vi "simplePID core.vi"(0 "errors":T2 {"error" step=0.125}, 1 "reset? (F)":bool, 7 "manual control":T6, 11 "state in":T3, 12 "gains":T4 {"filter coefficient" min=0 max=1; "proportional gain" step=0.125}, 13 "output range":T5={"output high (Inf)"=inf, "output low (-Inf)"=-inf}) -> (4 "output":sgl, 6 "error":sgl, 8 "actions":T1, 15 "state out":T3)   [LabVIEW 2020]
uses:
  Typedef/niFpgaPID_ManualControl.ctl
  Typedef/niFpgaPID_OutputRange.ctl
  Typedef/niFpgaPID_PIDGains.ctl
  <vilib>/rvi/Analysis/control/PID/Typedef/niFpgaPID_PIDState.ctl
  <vilib>/rvi/Analysis/control/PID/Typedef/niFpgaPID_PIDErrors.ctl
  Typedef/niFpgaPID_PIDActions.ctl
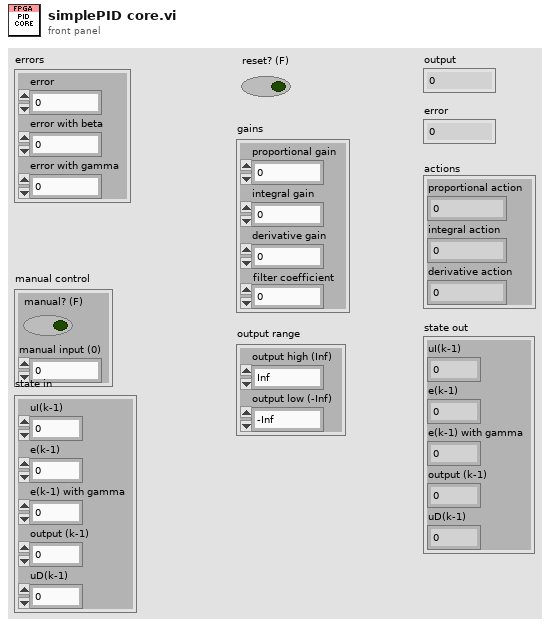
[diagram p1: front panel]
types:
  T1 = typedef "niFpgaPID_PIDActions.ctl" = cluster{"proportional action":sgl, "integral action":sgl, "derivative action":sgl}
  T2 = typedef "niFpgaPID_PIDErrors.ctl" = cluster{"error":sgl, "error with beta":sgl, "error with gamma":sgl}
  T3 = typedef "niFpgaPID_PIDState.ctl" = cluster{"uI(k-1)":sgl, "e(k-1)":sgl, "e(k-1) with gamma":sgl, "output (k-1)":sgl, "uD(k-1)":sgl}
  T4 = typedef "niFpgaPID_PIDGains.ctl" = cluster{"proportional gain":sgl, "integral gain":sgl, "derivative gain":sgl, "filter coefficient":sgl}
  T5 = typedef "niFpgaPID_OutputRange.ctl" = cluster{"output high (Inf)":sgl, "output low (-Inf)":sgl}
  T6 = typedef "niFpgaPID_ManualControl.ctl" = cluster{"manual? (F)":bool, "manual input (0)":sgl}
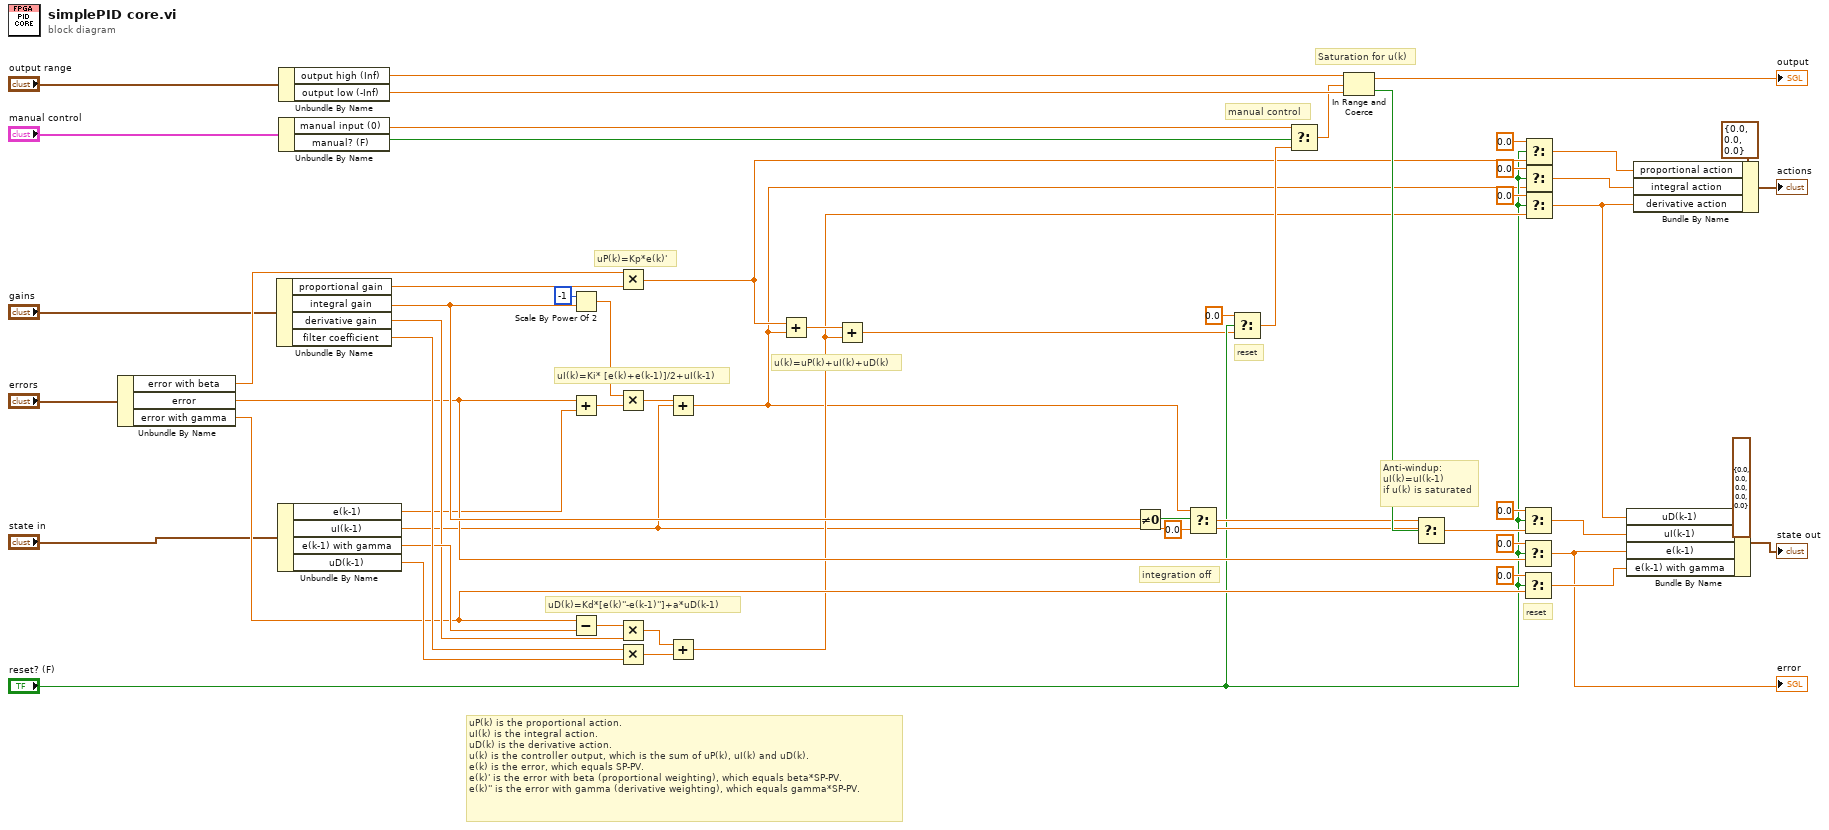
[diagram p0: block diagram]
diagram:
  # "uP(k) is the proportional action.\nuI(k) is the integral action.\nuD(k) is the derivative action.\nu(k) is the controller output, which is the sum of uP(k), uI(k) and uD(k).\ne(k) is the error, which equals SP-PV.\ne(k)' is the error with beta (proportional weighting), which equals beta*SP-PV.\ne(k)'' is the error with gamma (derivative weighting), which equals gamma*SP-PV."
  # "manual control"
  # "reset"
  # "reset"
  # "integration off"
  # "u(k)=uP(k)+uI(k)+uD(k)"
  # "uI(k)=Ki* [e(k)+e(k-1)]/2+uI(k-1)"
  # "uD(k)=Kd*[e(k)''-e(k-1)'']+a*uD(k-1)"
  # "uP(k)=Kp*e(k)'"
  # "Anti-windup:\nuI(k)=uI(k-1) \nif u(k) is saturated"
  # "Saturation for u(k)"
  n1 = Unbundle By Name("errors") -> ("error with beta"=w46:sgl, "error"=w27:sgl, "error with gamma"=w25:sgl)
  n2 = Unbundle By Name("gains") -> ("proportional gain"=w47:sgl, "integral gain"=w38:sgl, "derivative gain"=w40:sgl, "filter coefficient"=w52:sgl)
  n3 = Unbundle By Name("state in") -> ("e(k-1)"=w14:sgl, "uI(k-1)"=w13:sgl, "e(k-1) with gamma"=w45:sgl, "uD(k-1)"=w51:sgl)
  n4 = Unbundle By Name("output range") -> ("output high (Inf)"=w57:sgl, "output low (-Inf)"=w56:sgl)
  n5 = Unbundle By Name("manual control") -> ("manual input (0)"=w37:sgl, "manual? (F)"=w36:bool)
  n6 = Scale By Power Of 2(n=i16 -1, x=w38) -> (x*2^n=w42:sgl)
  n7 = Add(x=w27, y=w14) -> (x+y=w43:sgl)
  n8 = Subtract(x=w25, y=w45) -> (x-y=w50:sgl)
  n9 = Multiply(x=w46, y=w47) -> (x*y=w16:sgl)
  n10 = Multiply(x=w42, y=w43) -> (x*y=w54:sgl)
  n11 = Multiply(x=w50, y=w40) -> (x*y=w49:sgl)
  n12 = Multiply(x=w52, y=w51) -> (x*y=w48:sgl)
  n13 = Add(x=w54, y=w13) -> (x+y=w1:sgl)
  n14 = Add(x=w49, y=w48) -> (x+y=w21:sgl)
  n15 = Add(x=w16, y=w1) -> (x+y=w53:sgl)
  n16 = Add(x=w53, y=w21) -> (x+y=w2:sgl)
  n17 = Not Equal To 0?(x=w38) -> (x != 0?=w39:bool)
  n18 = Select(t=w1, s=w39, f=sgl 0.0) -> (s? t:f=w34:sgl)
  n19 = Select(t=sgl 0.0, s="reset? (F)", f=w2) -> (s? t:f=w33:sgl)
  n20 = Select(t=w37, s=w36, f=w33) -> (s? t:f=w55:sgl)
  n21 = In Range and Coerce(upper limit=w57, x=w55, lower limit=w56) -> (coerced(x)=→"output":sgl, In Range?=w58:bool)
  n22 = Select(t=w34, s=w58, f=w13) -> (s? t:f=w29:sgl)
  n23 = Select(t=sgl 0.0, s="reset? (F)", f=w29) -> (s? t:f=w30:sgl)
  n24 = Select(t=sgl 0.0, s="reset? (F)", f=w27) -> (s? t:f=w3:sgl)
  "error" <- w3
  n25 = Select(t=sgl 0.0, s="reset? (F)", f=w25) -> (s? t:f=w24:sgl)
  n26 = Select(t=sgl 0.0, s="reset? (F)", f=w16) -> (s? t:f=w17:sgl)
  n27 = Select(t=sgl 0.0, s="reset? (F)", f=w1) -> (s? t:f=w15:sgl)
  n28 = Select(t=sgl 0.0, s="reset? (F)", f=w21) -> (s? t:f=w20:sgl)
  n29 = Bundle By Name(cluster=T3 {"uI(k-1)"=0.0, "e(k-1)"=0.0, "e(k-1) with gamma"=0.0, "output (k-1)"=0.0, "uD(k-1)"=0.0} ("state"), "uD(k-1)"=w20, "uI(k-1)"=w30, "e(k-1)"=w3, "e(k-1) with gamma"=w24) -> (→"state out":T3)
  n30 = Bundle By Name(cluster=T1 {"proportional action"=0.0, "integral action"=0.0, "derivative action"=0.0} ("actions"), "proportional action"=w17, "integral action"=w15, "derivative action"=w20) -> (→"actions":T1)
